vi "GV trigger.vi"() -> ()   [LabVIEW 2017]
panel:
  in  "Trigger":bool
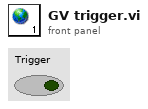
[diagram p1: front panel]
diagram:
